vi "DefineLink.vi"(2 "String":string) -> (4 "String 2":string)   [LabVIEW 2010]
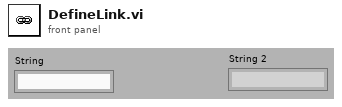
[diagram p1: front panel]
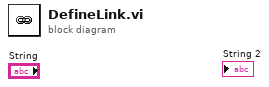
[diagram p0: block diagram]
diagram:
